vi "Create Client.vi"(8 "error in":errorcluster) -> (0 "error out":errorcluster, 3 "Client out":refnum<class "Client.lvclass">)   [LabVIEW 2020, in "Client.lvlib"]
doc: "Create a PVAccess client."
uses:
  Client.lvlib
  Client/Client.lvclass
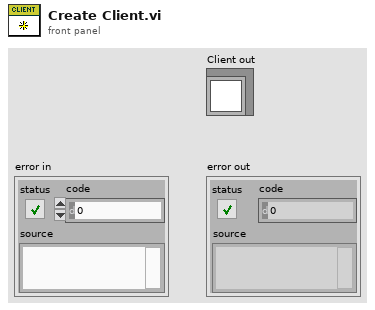
[diagram p1: front panel]
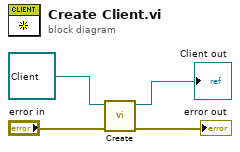
[diagram p0: block diagram]
diagram:
  n1 = call "Create.vi"("error in (no error)"="error in", "Client in"=refnum<class "Client.lvclass"> refnum ("Untitled Library 1:Client.lvclass")) -> ("error out"=→"error out":errorcluster, "Client out"=→"Client out":refnum<class "Client.lvclass">)  [unwired: 8 in]
